vi "LIVE PRICE.vi"() -> (2 "String 2":string, 3 "String":string)   [LabVIEW 2021]
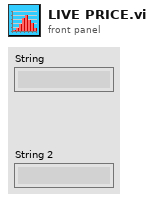
[diagram p1: front panel]
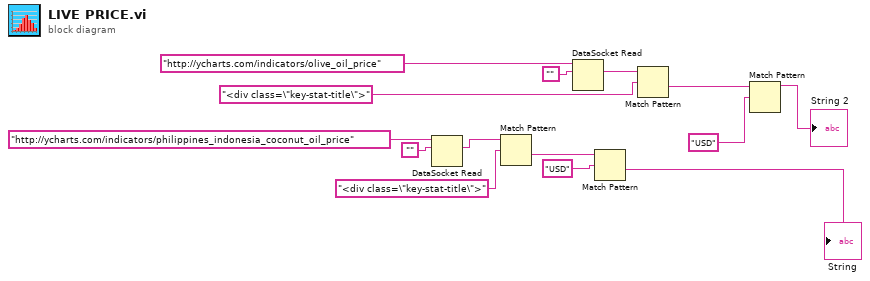
[diagram p0: block diagram]
diagram:
  n1 = DataSocket Read(10:"", 11:"http://ycharts.com/indicators/philippines_indonesia_coconut_oil_price" ("connection in")) -> (2:w14:string)  [unwired: 3 in, 6 out]
  n2 = Match Pattern(string=w14, regular expression="<div class=\"key-stat-title\">") -> (after substring=w2:string)  [unwired: 1 in, 3 out]
  n3 = DataSocket Read(10:"", 11:"http://ycharts.com/indicators/olive_oil_price") -> (2:w10:string)  [unwired: 3 in, 6 out]
  n4 = Match Pattern(string=w2, regular expression="USD") -> (before substring=→"String":string)  [unwired: 1 in, 3 out]
  n5 = Match Pattern(string=w10, regular expression="<div class=\"key-stat-title\">") -> (after substring=w8:string)  [unwired: 1 in, 3 out]
  n6 = Match Pattern(string=w8, regular expression="USD") -> (before substring=→"String 2":string)  [unwired: 1 in, 3 out]
